vi "Read Config File.vi"(8 "error in (no error)":cluster{"状态":bool, "代码":i32, "源":string} caption="错误输入（无错误）", 11 "气冷系统应用程序输入":refnum<class "Air Cooler Application.lvclass">) -> (0 "error out":cluster{"状态":bool, "代码":i32, "源":string} caption="错误输出", 3 "气冷系统应用程序输出":refnum<class "Air Cooler Application.lvclass">)   [LabVIEW 2013, in "Air Cooler Application.lvlib" / "Air Cooler Application.lvclass"]
doc: "本VI负责读取应用程序相关的配置文件，并将配置信息应用于应用程序对象。对于未在配置文件中找到的项，采用私有数据控件的默认值作为默认值。"
uses:
  Air Cooler Application.lvclass
  Air Cooler Application.lvclass/Air Cooler Application.ctl
  <vilib>/Utility/config.llb/NI_LVConfig.lvlib
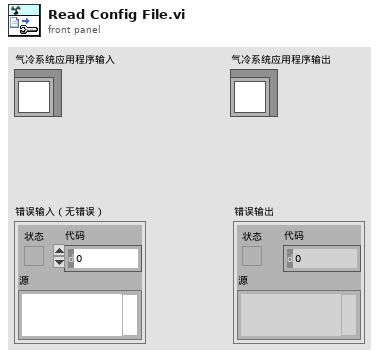
[diagram p1: front panel]
types:
  T1 = typedef "NI_LVConfig.lvlib/Config Data RefNum.ctl" = refnum<k1>
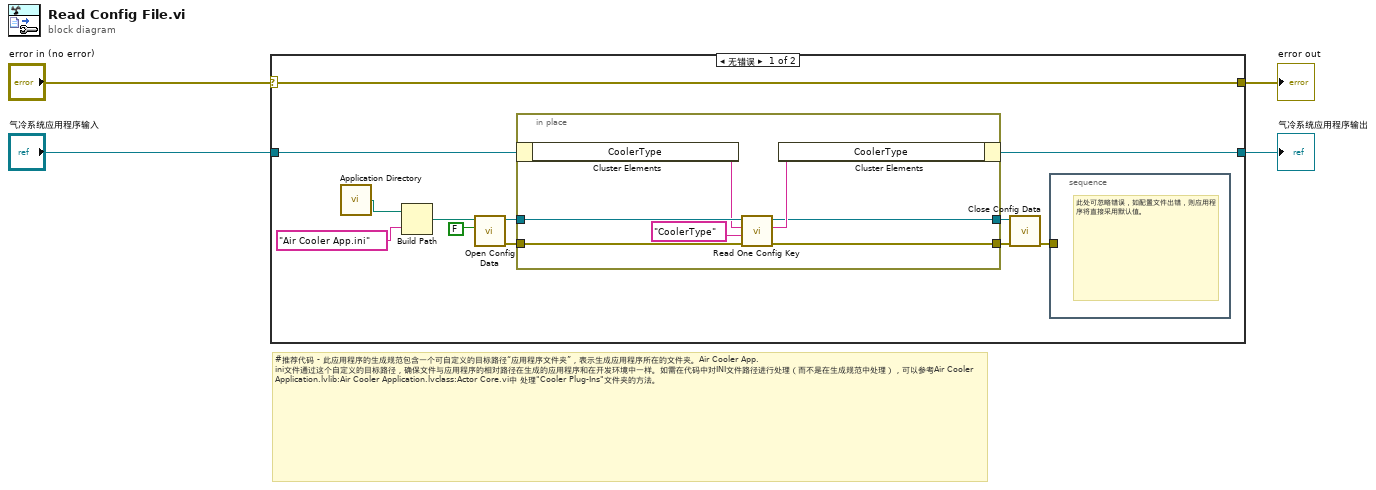
[diagram p0: block diagram]
diagram:
  # "#推荐代码 - 此应用程序的生成规范包含一个可自定义的目标路径“应用程序文件夹”，表示生成应用程序所在的文件夹。Air Cooler App.ini文件通过这个自定义的目标路径，确保文件与应用程序的相对路径在生成的应用程序和在开发环境中一样。如需在代码中对INI文件路径进行处理（而不是在生成规范中处理），可以参考Air Cooler Application.lvlib:Air Cooler Application.lvclass:Actor Core.vi中 处理\"Cooler Plug-Ins\"文件夹的方法。"
  n1 = case shown="无错误" "error in (no error)" {
    selector: "error in (no error)" -> [w10 w25]
    tunnel: [w10 w25] -> w3
    tunnel: [w8 w24] -> w1
    tunnel: "气冷系统应用程序输入" -> [w9 w24]
    frame No Error {
      n2 = call <vilib>:"Application Directory.vi"() -> ("Application Directory"=w16:path)
      n3 = Build Path(base path=w16, name or relative path="Air Cooler App.ini") -> (appended path=w5:path)
      n4 = call <vilib>:"Open Config Data.vi"("create file if necessary (T)"=FALSE, "configuration file path"=w5) -> ("error out"=w13:errorcluster, "refnum"=w12:T1)  [unwired: 7 in, 1 out]
      n5 = in-place {
        in-place-border: w13 -> [w23]
        in-place-border: w12 -> [w22]
        in-place-border: [w17] -> w7
        in-place-border: [w18] -> w6
        n6 = in-place-cluster #1(w9) -> ("CoolerType"=w19:string)
        n7 = call "Read One Config Key.vi"("error in (no error)"=w23, "键"="CoolerType" ("key"), "默认值"=w19, "引用句柄输入"=w22) -> ("error out"=w18:cluster{"状态":bool, "代码":i32, "源":string}, "值"=w20:string, "引用句柄输出"=w17:T1)  [unwired: 5 in]
        n8 = in-place-cluster #1("CoolerType"=w20) -> (w8:refnum<class "Air Cooler Application.lvclass">)
      }
      n9 = call <vilib>:"Close Config Data.vi"("error in (no error)"=w6, "refnum"=w7) -> ("error out"=w11:errorcluster)  [unwired: 8 in, 1 out]
      n10 = stacked-sequence {
        tunnel: w11 -> [_]
        frame #0 {
          # "此处可忽略错误，如配置文件出错，则应用程序将直接采用默认值。"
        }
      }
    }
    frame Error {
    }
  }
  "error out" <- w3
  "气冷系统应用程序输出" <- w1
